vi "Module Name--constant.vi"() -> (3 "Module Name":string)   [LabVIEW 2021, in "Configuration.lvlib"]
doc: "Return the name of the module that owns this VI. \n_____\nBased on DQMH Project Template 7.0.1.1316."
uses:
  Configuration.lvlib
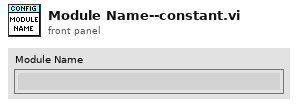
[diagram p1: front panel]
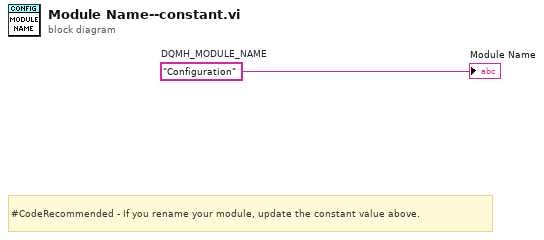
[diagram p0: block diagram]
diagram:
  w1 = "Configuration"  # DQMH_MODULE_NAME
  # "#CodeRecommended - If you rename your module, update the constant value above."
  "Module Name" <- w1
